vi "Dashboard Loop.vi"(11 "connection ID":refnum<k16>) -> ()   [LabVIEW 2016]
uses:
  Common Code/Dashboard Display Data.ctl
  Common Code/Climb Status Cluster.ctl
  Common Code/Drivetrain Status Cluster.ctl
  Common Code/Intake Status Cluster.ctl
  Common Code/Intake Modes.ctl
  Common Code/Intake Auto States.ctl
  Common Code/Intake Trip States.ctl
  Common Code/Shooter Status Cluster.ctl
  Common Code/Shooter Modes.ctl
  Common Code/Shot Type.ctl
  Common Code/Shooter Commands.ctl
  Common Code/Drivetrain Encoder Values.ctl
  Common Code/Encoder Values.ctl
  Common Code/Auton Command Cluster.ctl
  Common Code/Auton File Lists.ctl
  Common Code/Shooter Motor Operational Status .ctl
  Robot Global Data.vi
panel:
  out "Length":dbl
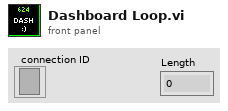
[diagram p1: front panel]
types:
  T1 = typedef "Dashboard Display Data.ctl" = cluster{"Climb Status Cluster":T2, "Drivetrain Status Cluster":T3, "Intake Status Cluster":T4, "Shooter Status Cluster":T8, "Drivetrain Encoder Values":T12, "Auton Command Cluster":T14, "Auton File Lists":T15, "Pressure":dbl, "Pressure Voltage":dbl, "Motor Operational Status":T16}
  T2 = typedef "Climb Status Cluster.ctl" = cluster{"Climb Speed":dbl}
  T3 = typedef "Drivetrain Status Cluster.ctl" = cluster{"Drivetrain Mode":enum16{"Manual", "Gyro Steer"}, "Y (Throttle)":dbl, "X (Steer)":dbl, "Z (Strafe)":dbl, "Heading Target":dbl, "Center Piston Down?":bool, "Traction?":bool, "Gyro Steer Finished?":bool, "Distance Drive Finished?":bool, "Gyro":dbl, "Distance Target":dbl, "Y Max Output":dbl, "Y Min Output":dbl, "X Max Output":dbl, "X Min Output":dbl, "Z Max Output":dbl, "Z Min Output":dbl, "Translation Target":dbl, "Translation Drive Finished?":bool, "PID Auto Drive Finished?":bool, "Brake?":bool, "Vision Aligned?":bool, "Creep Mode Engaged?":bool}
  T4 = typedef "Intake Status Cluster.ctl" = cluster{"Roller Power":dbl, "Intake Mode":T5, "Intake Auto State":T6, "Backward Tripped?":bool, "Forward Tripped?":bool, "Intake Current Trip State":T7, "Gear Slot Open":bool, "Wings Open":bool, "Traction for Gear?":bool}
  T5 = typedef "Intake Modes.ctl" = enum16{"Manual", "Auto"}
  T6 = typedef "Intake Auto States.ctl" = enum16{"Outake Ball", "Idle", "Load Ball"}
  T7 = typedef "Intake Trip States.ctl" = enum16{"Normal", "Backward Tripped", "Forward Tripped"}
  T8 = typedef "Shooter Status Cluster.ctl" = cluster{"Current RPM":dbl, "Trigger Power":dbl, "Shooter Mode":T9, "Shot Type":T10, "Shooter State":T11, "Target RPM":dbl, "Hood Down?":bool, "RPM Reached?":bool}
  T9 = typedef "Shooter Modes.ctl" = enum16{"Auto", "Manual"}
  T10 = typedef "Shot Type.ctl" = enum16{"Dist Shot", "Key Shot"}
  T11 = typedef "Shooter Commands.ctl" = enum16{"Idle ", "Warmup ", "Shoot"}
  T12 = typedef "Drivetrain Encoder Values.ctl" = cluster{"Left Encoder":T13, "Center Encoder":T13, "Right Encoder":T13}
  T13 = typedef "Encoder Values.ctl" = cluster{"Distance":dbl, "Speed":dbl, "Tick":dbl}
  T14 = typedef "Auton Command Cluster.ctl" = cluster{"commandID":dbl, "maxTime":dbl, "distanceTarget":dbl, "headingTarget":dbl, "translationTarget":dbl, "ySpeed":dbl, "xSpeed":dbl, "zSpeed":dbl, "async":dbl, "RPM":dbl, "Hood?":dbl, "Hopper?":dbl, "rollerPower":dbl, "fillHopper?":dbl, "zeroGyro":dbl, "openGear":dbl}
  T15 = typedef "Auton File Lists.ctl" = cluster{"Current Queue":string, "General Scripts":string, "Movements":string}
  T16 = typedef "Shooter Motor Operational Status .ctl" = cluster{"Sensor Velocity ":dbl, "Encoder Position":dbl, "Encoder Velocity ":dbl, "Encoder Index Count":dbl, "Analog In":dbl, "Analog In Velocity":dbl, "Battery Voltage":dbl, "Current":dbl, "Sensor Position":dbl, "Vel Div 4":bool, "Encoder A Pin State":bool, "Encoder B Pin State":bool, "Encoder Index Pin State":bool, "Pulse Width Velocity ":dbl}
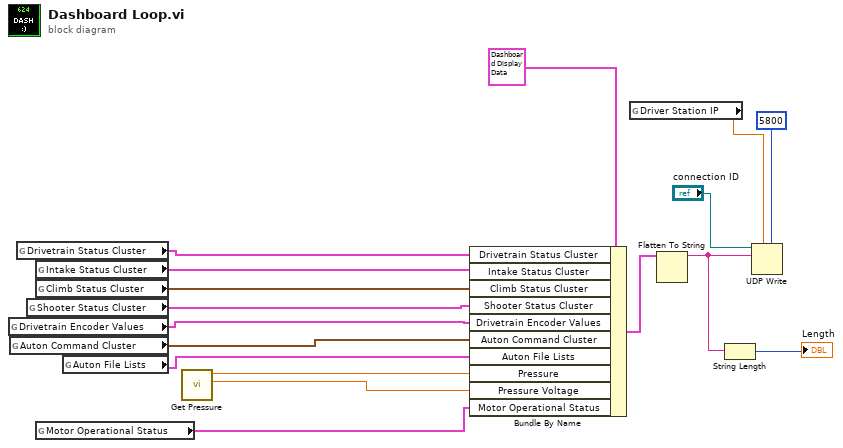
[diagram p0: block diagram]
diagram:
  n1 = global read "Robot Global Data.vi" "Drivetrain Encoder Values"() -> (w6:T12)
  n2 = global read "Robot Global Data.vi" "Auton Command Cluster"() -> (w5:T14)
  n3 = global read "Robot Global Data.vi" "Drivetrain Status Cluster"() -> (w10:T3)
  n4 = global read "Robot Global Data.vi" "Shooter Status Cluster"() -> (w7:T8)
  n5 = global read "Robot Global Data.vi" "Intake Status Cluster"() -> (w9:T4)
  n6 = global read "Robot Global Data.vi" "Climb Status Cluster"() -> (w8:T2)
  n7 = global read "Robot Global Data.vi" "Motor Operational Status"() -> (w1:T16)
  n8 = global read "Robot Global Data.vi" "Auton File Lists"() -> (w4:T15)
  n9 = call "Get Pressure.vi"() -> ("Pressure Voltage"=w2:dbl, "Pressure"=w3:dbl)  [unwired: 10 in]
  n10 = Bundle By Name(cluster=T1 {"Climb Status Cluster"={"Climb Speed"=0.0}, "Drivetrain Status Cluster"={"Drivetrain Mode"=enum."Manual", "Y (Throttle)"=0.0, "X (Steer)"=0.0, "Z (Strafe)"=0.0, "Heading Target"=0.0, "Center Piston Down?"=FALSE, "Traction?"=FALSE, "Gyro Steer Finished?"=FALSE, "Distance Drive Finished?"=FALSE, "Gyro"=0.0, "Distance Target"=0.0, "Y Max Output"=0.0, "Y Min Output"=0.0, "X Max Output"=0.0, "X Min Output"=0.0, "Z Max Output"=0.0, "Z Min Output"=0.0, "Translation Target"=0.0, "Translation Drive Finished?"=FALSE, "PID Auto Drive Finished?"=FALSE, "Brake?"=FALSE, "Vision Aligned?"=FALSE, "Creep Mode Engaged?"=FALSE}, "Intake Status Cluster"={"Roller Power"=0.0, "Intake Mode"=enum."Manual", "Intake Auto State"=enum."Idle", "Backward Tripped?"=FALSE, "Forward Tripped?"=FALSE, "Intake Current Trip State"=enum."Normal", "Gear Slot Open"=FALSE, "Wings Open"=FALSE, "Traction for Gear?"=FALSE}, "Shooter Status Cluster"={"Current RPM"=0.0, "Trigger Power"=0.0, "Shooter Mode"=enum."Auto", "Shot Type"=enum."Dist Shot", "Shooter State"=enum."Idle ", "Target RPM"=0.0, "Hood Down?"=FALSE, "RPM Reached?"=FALSE}, "Drivetrain Encoder Values"={"Left Encoder"={"Distance"=0.0, "Speed"=0.0, "Tick"=0.0}, "Center Encoder"={"Distance"=0.0, "Speed"=0.0, "Tick"=0.0}, "Right Encoder"={"Distance"=0.0, "Speed"=0.0, "Tick"=0.0}}, "Auton Command Cluster"={"commandID"=0.0, "maxTime"=0.0, "distanceTarget"=0.0, "headingTarget"=0.0, "translationTarget"=0.0, "ySpeed"=0.0, "xSpeed"=0.0, "zSpeed"=0.0, "async"=0.0, "RPM"=0.0, "Hood?"=0.0, "Hopper?"=0.0, "rollerPower"=0.0, "fillHopper?"=0.0, "zeroGyro"=0.0, "openGear"=0.0}, "Auton File Lists"={"Current Queue"="", "General Scripts"="", "Movements"=""}, "Pressure"=0.0, "Pressure Voltage"=0.0, "Motor Operational Status"={"Sensor Velocity "=0.0, "Encoder Position"=0.0, "Encoder Velocity "=0.0, "Encoder Index Count"=0.0, "Analog In"=0.0, "Analog In Velocity"=0.0, "Battery Voltage"=0.0, "Current"=0.0, "Sensor Position"=0.0, "Vel Div 4"=FALSE, "Encoder A Pin State"=FALSE, "Encoder B Pin State"=FALSE, "Encoder Index Pin State"=FALSE, "Pulse Width Velocity "=0.0}} ("Dashboard Display Data"), "Drivetrain Status Cluster"=w10, "Intake Status Cluster"=w9, "Climb Status Cluster"=w8, "Shooter Status Cluster"=w7, "Drivetrain Encoder Values"=w6, "Auton Command Cluster"=w5, "Auton File Lists"=w4, "Pressure"=w3, "Pressure Voltage"=w2, "Motor Operational Status"=w1) -> (w13:T1)
  n11 = global read "Robot Global Data.vi" "Driver Station IP"() -> (w11:dbl)
  n12 = Flatten To String(anything=w13) -> (data string=w15:string)  [unwired: 3 in, 2 out]
  n13 = String Length(string=w15) -> (length=→"Length":i32)
  n14 = UDP Write(address=w11, port or service name=5800, connection ID="connection ID", data in=w15) -> ()  [unwired: 2 in, 2 out]
